vi "PDCGetAll.vi"(8 "error in (no error)":errorcluster, 10 "ChildNo":u32, 11 "DeviceNo":u32) -> (0 "error out":errorcluster)   [LabVIEW 2015]
panel:
  out "ResolutionList":string[](array[string])
  out "BitDepth":i8
  out "ColorType":i8
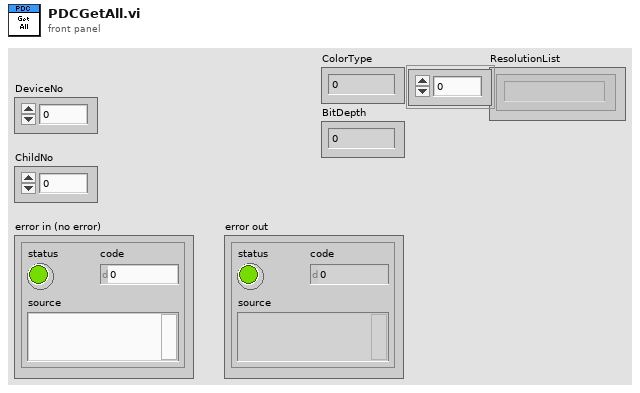
[diagram p1: front panel]
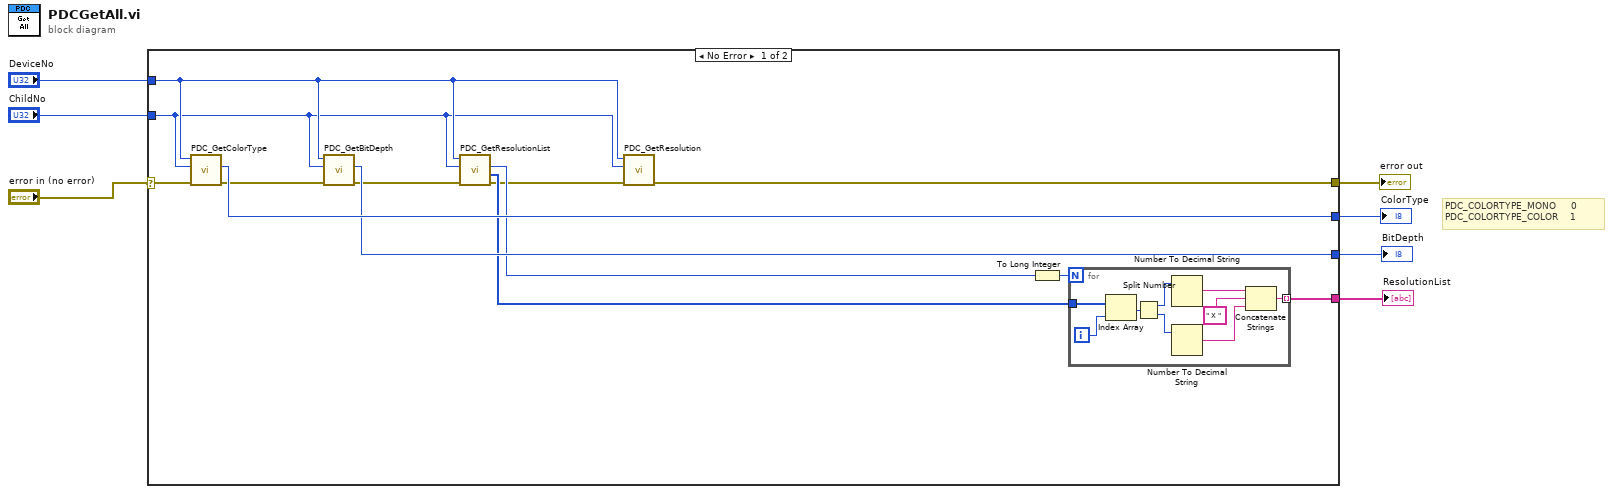
[diagram p0: block diagram]
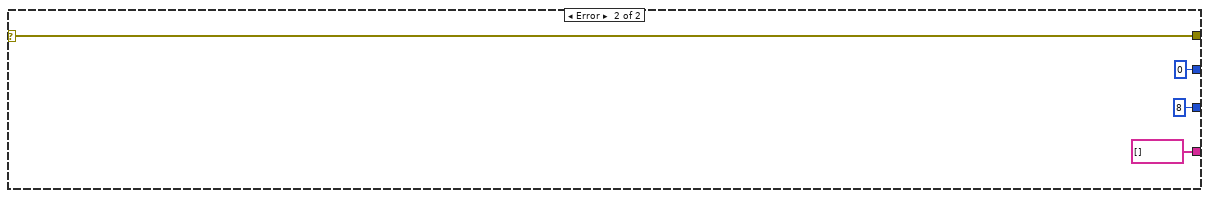
[diagram p2: hidden frame]
diagram:
  # "PDC_COLORTYPE_MONO\t\t\t\t\t0\nPDC_COLORTYPE_COLOR\t\t\t\t1"
  n1 = case shown="No Error" "error in (no error)" {
    selector: "error in (no error)" -> [w20 w33]
    tunnel: [w10 w33] -> w7
    tunnel: "ChildNo" -> [w8 _]
    tunnel: "DeviceNo" -> [w9 _]
    tunnel: [w19 i8 0 ("Mode")] -> w3
    tunnel: [w17 i8 8 ("Depth")] -> w2
    tunnel: [w15 string[] []] -> w1
    frame No Error {
      n2 = call "PDC_GetColorType.vi"("error in (no error)"=w20, "ChildNo"=w8, "DeviceNo"=w9) -> ("error out"=w18:errorcluster, "Mode"=w19:i8)  [unwired: 5 in, 2 out]
      n3 = call "PDC_GetBitDepth.vi"("error in (no error)"=w18, "ChildNo"=w8, "DeviceNo"=w9) -> ("error out"=w16:errorcluster, "Depth"=w17:i8)  [unwired: 5 in, 2 out]
      n4 = call "PDC_GetResolutionList.vi"("error in (no error)"=w16, "ChildNo"=w8, "DeviceNo"=w9) -> ("error out"=w11:errorcluster, "List"=w14:u32[], "Size"=w12:u32)  [unwired: 4 in, 2 out]
      n5 = call "PDC_GetResolution.vi"("error in (no error)"=w11, "ChildNo"=w8, "DeviceNo"=w9) -> ("error out"=w10:errorcluster)  [unwired: 4 in, 4 out]
      n6 = To Long Integer(number=w12) -> (32bit integer=w13:i32)
      n7 = for {
        N: w13 -> [_]
        tunnel: [w27] -> w15 mode=indexing
        tunnel: w14 -> [w26]
        i -> [w25]
        n8 = Index Array(array=w26, index=w25) -> (element=w24:u32)
        n9 = Split Number(x=w24) -> (hi(x)=w23:u16, lo(x)=w22:u16)
        n10 = Number To Decimal String(number=w23) -> (decimal integer string=w29:string)  [unwired: 1 out]
        n11 = Number To Decimal String(number=w22) -> (decimal integer string=w28:string)  [unwired: 1 out]
        n12 = Concatenate Strings(w29, " X ", w28) -> (w27:string)
      }
    }
    frame Error {
    }
  }
  "error out" <- w7
  "ColorType" <- w3
  "BitDepth" <- w2
  "ResolutionList" <- w1
